vi "getStatus.vi"(8 "error in (no error)":errorcluster, 11 "DS360 in":refnum<class "DS360.lvclass">) -> (0 "error out":errorcluster, 2 "read buffer":string, 3 "DS360 out":refnum<class "DS360.lvclass">)   [LabVIEW 2019, in "DS360.lvclass"]
uses:
  DS360.lvclass
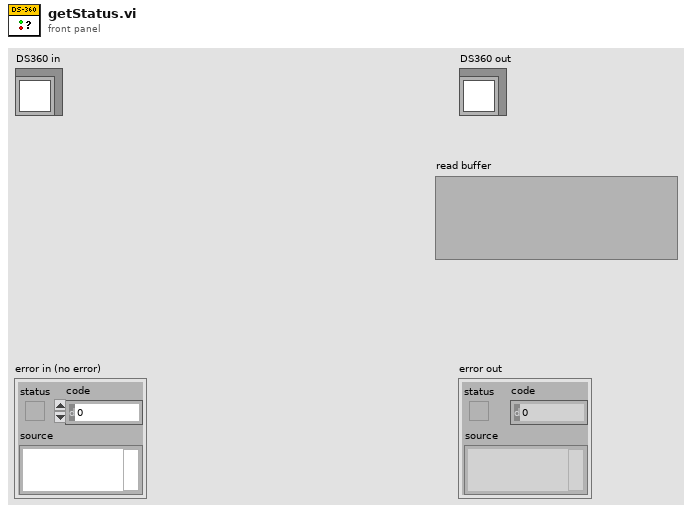
[diagram p1: front panel]
types:
  T1 = cluster{"error":bool, "code":i32, "source":string}
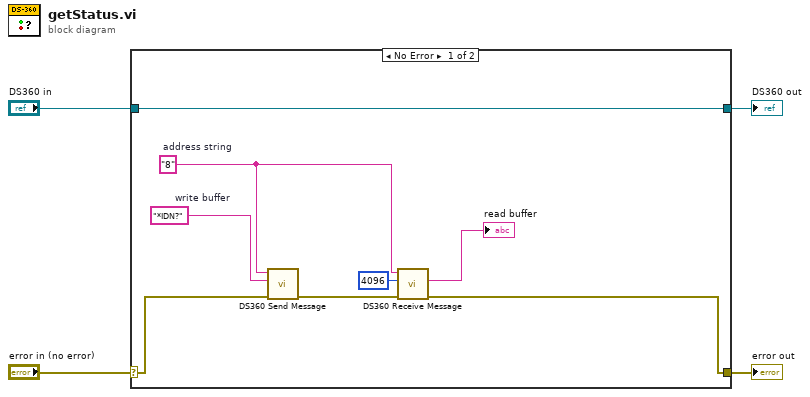
[diagram p0: block diagram]
diagram:
  n1 = case shown="No Error" "error in (no error)" {
    selector: "error in (no error)" -> [w6 w14]
    tunnel: [w5 w14] -> w3
    tunnel: [w12 w13] -> w1
    tunnel: "DS360 in" -> [w12 w13]
    frame No Error {
      w11 = "*IDN?"  # write buffer
      w9 = "8"  # address string
      n2 = call <instrlib>:"DS360 Send Message.vi"("address string"=w9, "write buffer"=w11, "error in"=w6) -> ("error out"=w10:T1)  [unwired: 3 in, 3 out]
      n3 = call <instrlib>:"DS360 Receive Message.vi"("address string"=w9, "byte count"=4096, "error in"=w10) -> ("read buffer"=→"read buffer":string, "error out"=w5:T1)  [unwired: 3 in, 2 out]
    }
    frame Error {
    }
  }
  "error out" <- w3
  "DS360 out" <- w1
